vi "Bus Monitor Suite.vi"   [LabVIEW 2020, in "Unit Tests.lvlib"]
uses:
  Unit Tests.lvlib
  Tests/Bus Monitor/Bus Monitor.lvclass
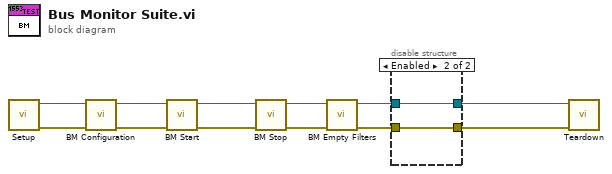
[diagram p0: block diagram]
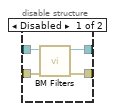
[diagram p2: hidden frame]
diagram:
  n1 = call "Setup.vi"() -> ("error out"=w11:errorcluster, "Bus Monitor out"=w12:refnum<class "Bus Monitor.lvclass">)  [unwired: 10 in]
  n2 = call "BM Configuration.vi"("error in (no error)"=w11, "Bus Monitor in"=w12) -> ("error out"=w2:errorcluster, "Bus Monitor out"=w1:refnum<class "Bus Monitor.lvclass">)  [unwired: 8 in]
  n3 = call "BM Start.vi"("error in (no error)"=w2, "Bus Monitor in"=w1) -> ("error out"=w4:errorcluster, "Bus Monitor out"=w3:refnum<class "Bus Monitor.lvclass">)  [unwired: 8 in]
  n4 = call "BM Stop.vi"("error in (no error)"=w4, "Bus Monitor in"=w3) -> ("error out"=w6:errorcluster, "Bus Monitor out"=w5:refnum<class "Bus Monitor.lvclass">)  [unwired: 8 in]
  n5 = call "BM Empty Filters.vi"("error in (no error)"=w6, "Bus Monitor in"=w5) -> ("error out"=w8:errorcluster, "Bus Monitor out"=w7:refnum<class "Bus Monitor.lvclass">)  [unwired: 8 in]
  n6 = disable-structure shown="Enabled" {
    disable-tunnel: w8 -> [w16 w17]
    disable-tunnel: w7 -> [w15 w18]
    disable-tunnel: [w14 w18] -> w10
    disable-tunnel: [w13 w17] -> w9
    frame Disabled {
      n7 = call "BM Filters.vi"("error in (no error)"=w16, "Bus Monitor in"=w15) -> ("error out"=w13:errorcluster, "Bus Monitor out"=w14:refnum<class "Bus Monitor.lvclass">)  [unwired: 8 in]
    }
    frame Enabled {
    }
  }
  n8 = call "Teardown.vi"("error in (no error)"=w9, "Bus Monitor in"=w10) -> ()  [unwired: 9 in, 1 out]
